vi "S2C_VLFT10_Proc_Commands.vi"(7 "VI_Ref":refnum<vi>, 8 "Error In":errorcluster, 10 "Settings":T1, 11 "Q-Ref":refnum<queue>) -> (0 "Error Out":errorcluster, 2 "Exit?":bool, 3 "Response":variant)   [LabVIEW 2015]
uses:
  S2C_VLFT10_Proc_Globals.vi
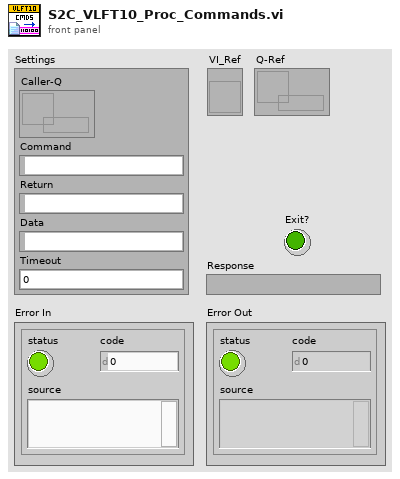
[diagram p1: front panel]
types:
  T1 = cluster{"Caller-Q":refnum<queue>, "Command":string, "Return":string, "Data":variant, "Timeout":dbl}
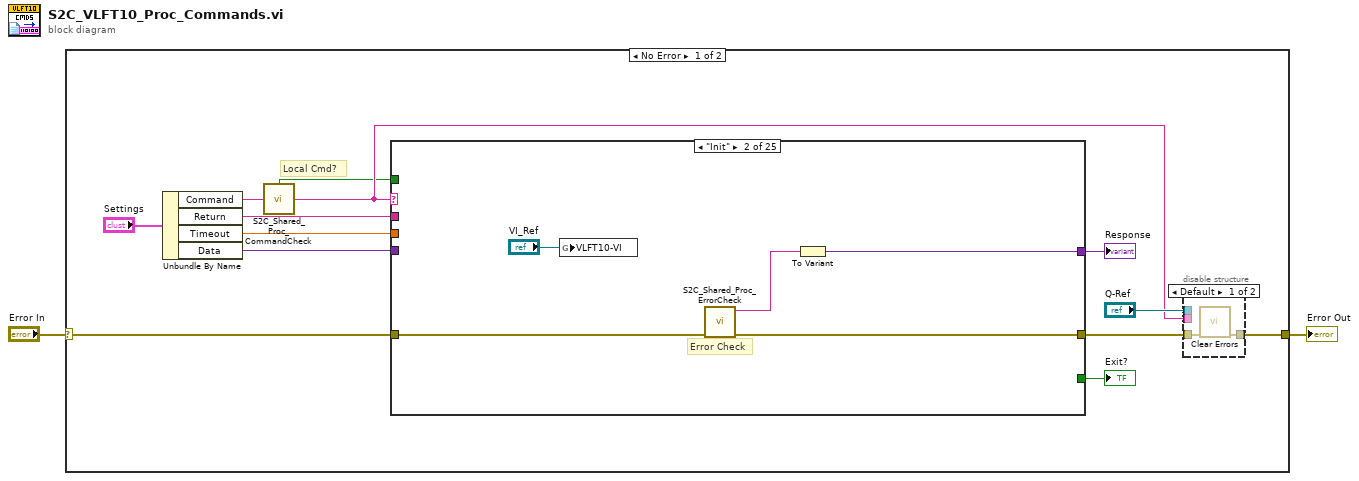
[diagram p0: block diagram]
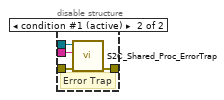
[diagram p2: hidden frame]
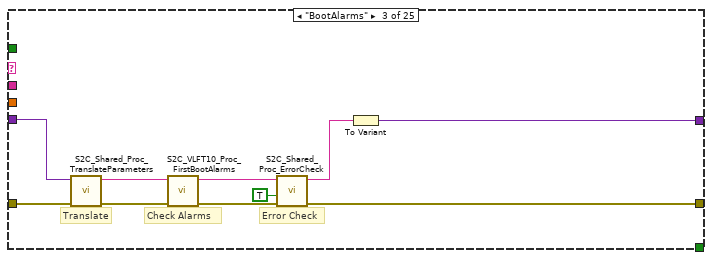
[diagram p4: hidden frame]
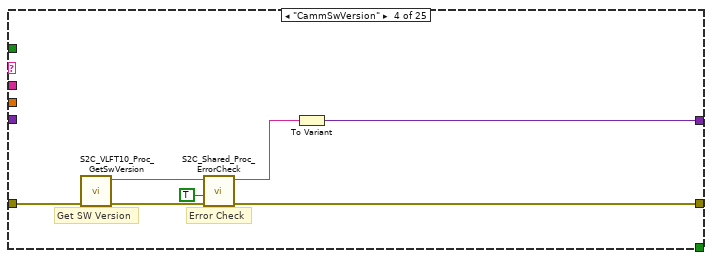
[diagram p5: hidden frame]
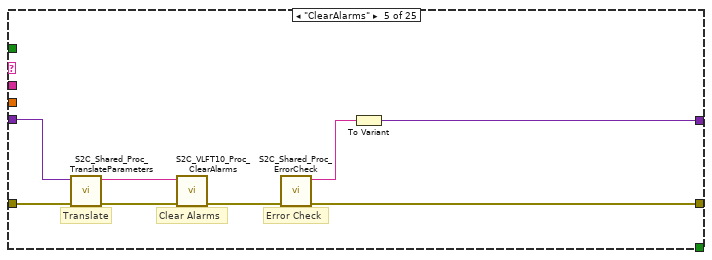
[diagram p6: hidden frame]
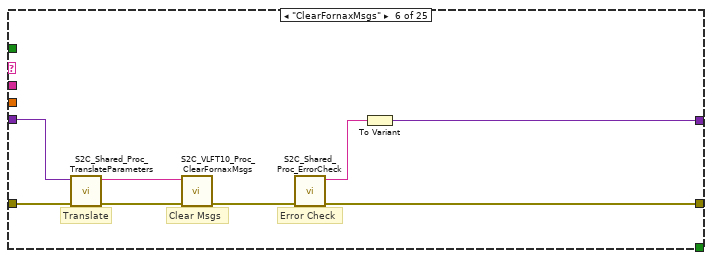
[diagram p7: hidden frame]
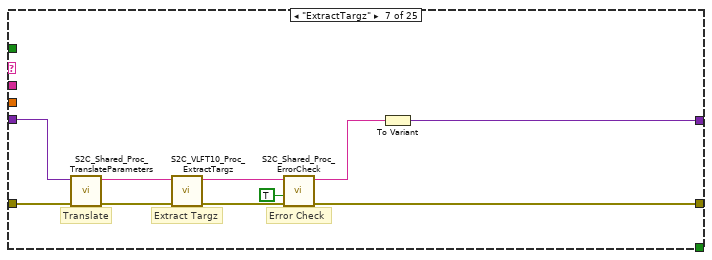
[diagram p8: hidden frame]
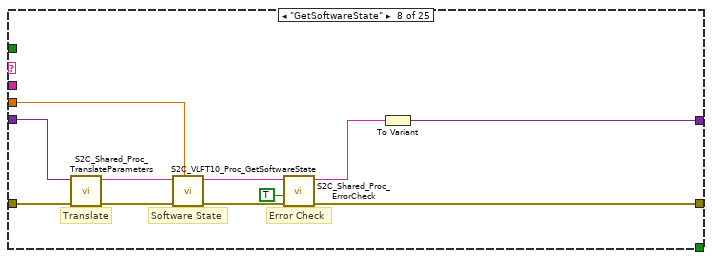
[diagram p9: hidden frame]
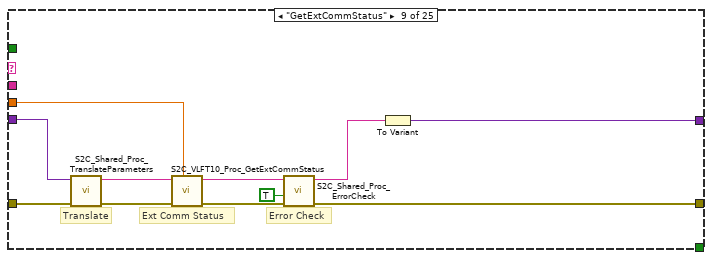
[diagram p10: hidden frame]
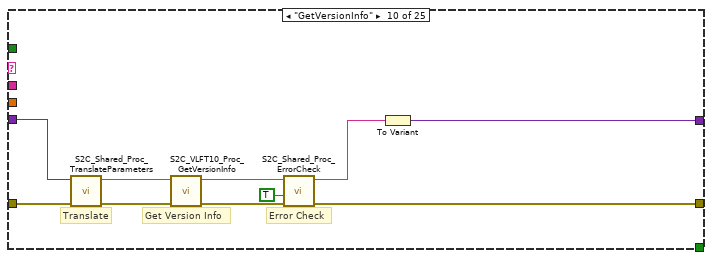
[diagram p11: hidden frame]
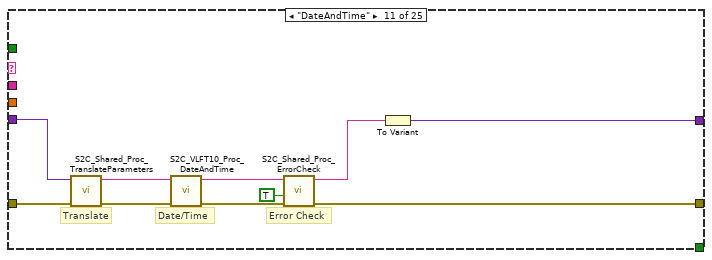
[diagram p12: hidden frame]
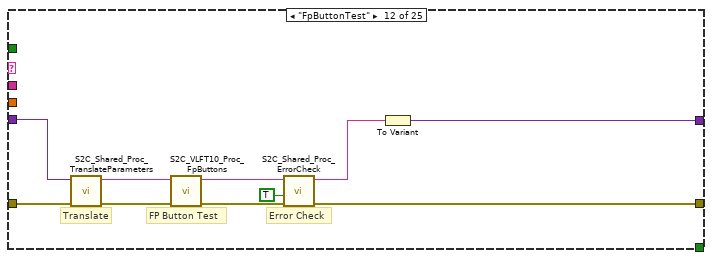
[diagram p13: hidden frame]
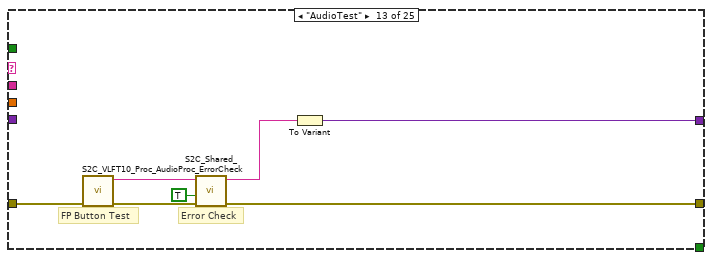
[diagram p14: hidden frame]
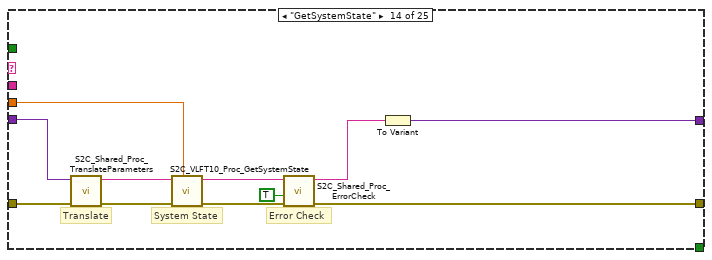
[diagram p15: hidden frame]
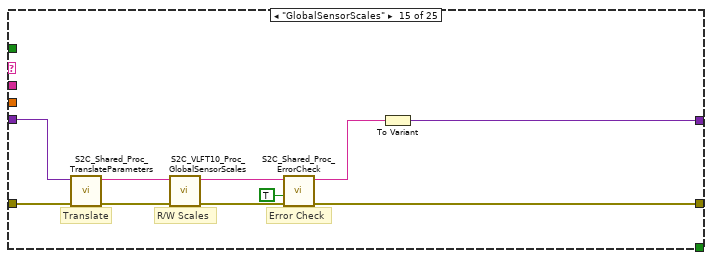
[diagram p16: hidden frame]
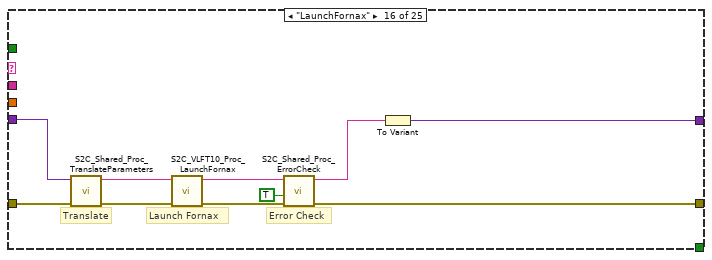
[diagram p17: hidden frame]
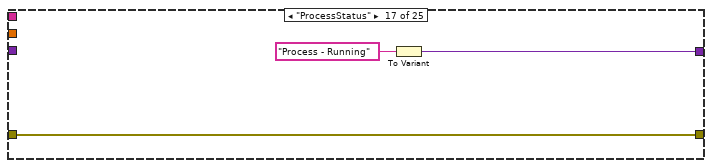
[diagram p18: hidden frame]
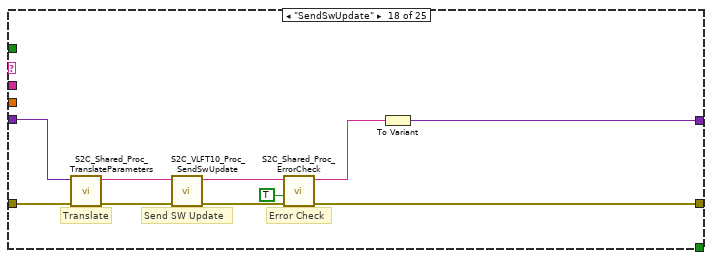
[diagram p19: hidden frame]
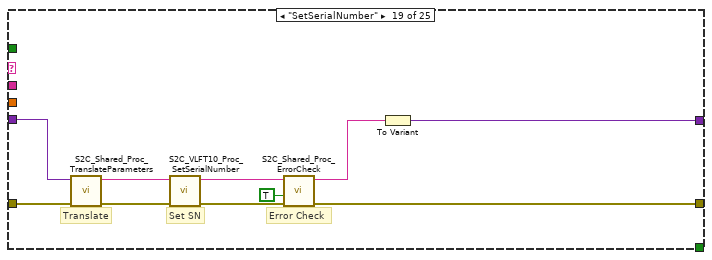
[diagram p20: hidden frame]
diagram:
  n1 = case shown="No Error" "Error In" {
    selector: "Error In" -> [w15 w237]
    tunnel: [w6 w236] -> w1
    frame No Error {
      # "Local Cmd?"
      n2 = Unbundle By Name("Settings") -> ("Command"=w5:string, "Return"=w12:string, "Timeout"=w10:dbl, "Data"=w11:variant)
      n3 = call "S2C_Shared_Proc_CommandCheck.vi"("Cmd In"=w5) -> ("Local?"=w3:bool, "Cmd Out"=w4:string)  [unwired: 13 in]
      n4 = case shown="\"Init\"" w4 {
        tunnel: w15 -> [w22 w23 w36 w39 w49 w57 w64 w75 w86 w96 w106 w116 w123 w134 w144 w154 w161 w167 w177 w187 w197 w208 w215 w225 w232]
        tunnel: [w22 w25 w28 w38 w50 w60 w65 w76 w87 w97 w107 w117 w124 w135 w145 w155 w161 w168 w178 w188 w198 w209 w216 w224 w227] -> w7
        tunnel: [_ w26 w37 w43 w51 w58 w70 w81 w92 w102 w112 w122 w129 w140 w150 w160 w163 w173 w183 w193 w203 w214 w221 _ w233] -> w14
        tunnel: w12 -> [_ _ _ _ _ _ _ _ _ _ _ _ _ _ _ _ _ _ _ _ _ _ _ _ _]
        tunnel: w11 -> [_ _ w35 _ w48 w53 w63 w74 w85 w95 w105 w115 _ w133 w143 w153 _ w166 w176 w186 w196 w207 _ w223 _]
        tunnel: w10 -> [_ _ _ _ _ _ _ w71 w82 _ _ _ _ w130 _ _ _ _ _ _ _ w204 _ _ _]
        tunnel: w3 -> [_ _ _ _ _ _ _ _ _ _ _ _ _ _ _ _ _ _ _ _ _ _ _ w222 _]
        tunnel: [_ _ _ _ _ _ _ _ _ _ _ _ _ _ _ _ _ _ _ _ _ _ _ _ TRUE] -> w9
        frame "Other", Default {
        }
        frame "Init" {
          # "Error Check"
          n5 = global write "S2C_VLFT10_Proc_Globals.vi" "VLFT10-VI"("VI_Ref") -> ()
          n6 = call "S2C_Shared_Proc_ErrorCheck.vi"("Error In"=w23) -> ("Error Out"=w25:errorcluster, "Status"=w27:string)  [unwired: 9 in]
          n7 = To Variant(anything=w27) -> (Variant=w26:variant)
        }
        frame "BootAlarms" {
          # "Check Alarms"
          # "Error Check"
          # "Translate"
          n8 = call "S2C_Shared_Proc_TranslateParameters.vi"("Error In"=w36, "Data"=w35) -> ("Error Out"=w30:errorcluster, "JSON Cluster"=w29:string)  [unwired: 8 in]
          n9 = call "S2C_VLFT10_Proc_FirstBootAlarms.vi"("Error In"=w30, "Exceptions"=w29) -> ("Error Out"=w33:errorcluster, "Pass?"=w32:string)  [unwired: 8 in]
          n10 = call "S2C_Shared_Proc_ErrorCheck.vi"("Error In"=w33, "ExpReply?"=TRUE, "Reply Text"=w32) -> ("Error Out"=w28:errorcluster, "Status"=w34:string)  [unwired: 7 in]
          n11 = To Variant(anything=w34) -> (Variant=w37:variant)
        }
        frame "CammSwVersion" {
          # "Get SW Version"
          # "Error Check"
          n12 = call "S2C_VLFT10_Proc_GetSwVersion.vi"("Error In"=w39) -> ("Error Out"=w42:errorcluster, "ItemValue"=w41:string)  [unwired: 8 in, 1 out]
          n13 = call "S2C_Shared_Proc_ErrorCheck.vi"("Error In"=w42, "ExpReply?"=TRUE, "Reply Text"=w41) -> ("Error Out"=w38:errorcluster, "Status"=w44:string)  [unwired: 7 in]
          n14 = To Variant(anything=w44) -> (Variant=w43:variant)
        }
        frame "ClearAlarms" {
          # "Clear Alarms"
          # "Translate"
          # "Error Check"
          n15 = call "S2C_Shared_Proc_TranslateParameters.vi"("Error In"=w49, "Data"=w48) -> ("Error Out"=w47:errorcluster, "JSON Cluster"=w45:string)  [unwired: 8 in]
          n16 = call "S2C_VLFT10_Proc_ClearAlarms.vi"("Error In"=w47, "Alarms"=w45) -> ("Error Out"=w46:errorcluster)  [unwired: 9 in]
          n17 = call "S2C_Shared_Proc_ErrorCheck.vi"("Error In"=w46) -> ("Error Out"=w50:errorcluster, "Status"=w52:string)  [unwired: 9 in]
          n18 = To Variant(anything=w52) -> (Variant=w51:variant)
        }
        frame "ClearFornaxMsgs" {
          # "Clear Msgs"
          # "Translate"
          # "Error Check"
          n19 = call "S2C_Shared_Proc_TranslateParameters.vi"("Error In"=w57, "Data"=w53) -> ("Error Out"=w56:errorcluster, "JSON Cluster"=w54:string)  [unwired: 8 in]
          n20 = call "S2C_VLFT10_Proc_ClearFornaxMsgs.vi"("Error In"=w56, "ClearMsg"=w54) -> ("Error Out"=w55:errorcluster)  [unwired: 9 in]
          n21 = call "S2C_Shared_Proc_ErrorCheck.vi"("Error In"=w55) -> ("Error Out"=w60:errorcluster, "Status"=w59:string)  [unwired: 9 in]
          n22 = To Variant(anything=w59) -> (Variant=w58:variant)
        }
        frame "ExtractTargz" {
          # "Translate"
          # "Extract Targz"
          # "Error Check"
          n23 = call "S2C_Shared_Proc_TranslateParameters.vi"("Error In"=w64, "Data"=w63) -> ("Error Out"=w62:errorcluster, "JSON Cluster"=w61:string)  [unwired: 8 in]
          n24 = call "S2C_VLFT10_Proc_ExtractTargz.vi"("Error In"=w62, "Paths"=w61) -> ("Error Out"=w68:errorcluster, "Result"=w67:string)  [unwired: 8 in]
          n25 = call "S2C_Shared_Proc_ErrorCheck.vi"("Error In"=w68, "ExpReply?"=TRUE, "Reply Text"=w67) -> ("Error Out"=w65:errorcluster, "Status"=w69:string)  [unwired: 7 in]
          n26 = To Variant(anything=w69) -> (Variant=w70:variant)
        }
        frame "GetSoftwareState" {
          # "Translate"
          # "Software State"
          # "Error Check"
          n27 = call "S2C_Shared_Proc_TranslateParameters.vi"("Error In"=w75, "Data"=w74) -> ("Error Out"=w73:errorcluster, "JSON Cluster"=w72:string)  [unwired: 8 in]
          n28 = call "S2C_VLFT10_Proc_GetSoftwareState.vi"("Timeout"=w71, "Error In"=w73, "State"=w72) -> ("Error Out"=w79:errorcluster, "Result"=w78:string)  [unwired: 7 in]
          n29 = call "S2C_Shared_Proc_ErrorCheck.vi"("Error In"=w79, "ExpReply?"=TRUE, "Reply Text"=w78) -> ("Error Out"=w76:errorcluster, "Status"=w80:string)  [unwired: 7 in]
          n30 = To Variant(anything=w80) -> (Variant=w81:variant)
        }
        frame "GetExtCommStatus" {
          # "Translate"
          # "Ext Comm Status"
          # "Error Check"
          n31 = call "S2C_Shared_Proc_TranslateParameters.vi"("Error In"=w86, "Data"=w85) -> ("Error Out"=w84:errorcluster, "JSON Cluster"=w83:string)  [unwired: 8 in]
          n32 = call "S2C_VLFT10_Proc_GetExtCommStatus.vi"("Timeout"=w82, "Error In"=w84, "Status"=w83) -> ("Error Out"=w90:errorcluster, "Result"=w89:string)  [unwired: 7 in]
          n33 = call "S2C_Shared_Proc_ErrorCheck.vi"("Error In"=w90, "ExpReply?"=TRUE, "Reply Text"=w89) -> ("Error Out"=w87:errorcluster, "Status"=w91:string)  [unwired: 7 in]
          n34 = To Variant(anything=w91) -> (Variant=w92:variant)
        }
        frame "GetVersionInfo" {
          # "Translate"
          # "Get Version Info"
          # "Error Check"
          n35 = call "S2C_Shared_Proc_TranslateParameters.vi"("Error In"=w96, "Data"=w95) -> ("Error Out"=w94:errorcluster, "JSON Cluster"=w93:string)  [unwired: 8 in]
          n36 = call "S2C_VLFT10_Proc_GetVersionInfo.vi"("Error In"=w94, "Item"=w93) -> ("Error Out"=w100:errorcluster, "Value"=w99:string)  [unwired: 7 in, 1 out]
          n37 = call "S2C_Shared_Proc_ErrorCheck.vi"("Error In"=w100, "ExpReply?"=TRUE, "Reply Text"=w99) -> ("Error Out"=w97:errorcluster, "Status"=w101:string)  [unwired: 7 in]
          n38 = To Variant(anything=w101) -> (Variant=w102:variant)
        }
        frame "DateAndTime" {
          # "Translate"
          # "Date/Time"
          # "Error Check"
          n39 = call "S2C_Shared_Proc_TranslateParameters.vi"("Error In"=w106, "Data"=w105) -> ("Error Out"=w104:errorcluster, "JSON Cluster"=w103:string)  [unwired: 8 in]
          n40 = call "S2C_VLFT10_Proc_DateAndTime.vi"("Error In"=w104, "Time"=w103) -> ("Error Out"=w110:errorcluster, "Result"=w109:string)  [unwired: 8 in]
          n41 = call "S2C_Shared_Proc_ErrorCheck.vi"("Error In"=w110, "ExpReply?"=TRUE, "Reply Text"=w109) -> ("Error Out"=w107:errorcluster, "Status"=w111:string)  [unwired: 7 in]
          n42 = To Variant(anything=w111) -> (Variant=w112:variant)
        }
        frame "FpButtonTest" {
          # "Translate"
          # "FP Button Test"
          # "Error Check"
          n43 = call "S2C_Shared_Proc_TranslateParameters.vi"("Error In"=w116, "Data"=w115) -> ("Error Out"=w114:errorcluster, "JSON Cluster"=w113:string)  [unwired: 8 in]
          n44 = call "S2C_VLFT10_Proc_FpButtons.vi"("Error In"=w114, "Button"=w113) -> ("Error Out"=w120:errorcluster, "Result"=w119:string)  [unwired: 8 in]
          n45 = call "S2C_Shared_Proc_ErrorCheck.vi"("Error In"=w120, "ExpReply?"=TRUE, "Reply Text"=w119) -> ("Error Out"=w117:errorcluster, "Status"=w121:string)  [unwired: 7 in]
          n46 = To Variant(anything=w121) -> (Variant=w122:variant)
        }
        frame "AudioTest" {
          # "FP Button Test"
          # "Error Check"
          n47 = call "S2C_VLFT10_Proc_Audio.vi"("Error In"=w123) -> ("Error Out"=w127:errorcluster, "Result"=w126:string)  [unwired: 9 in]
          n48 = call "S2C_Shared_Proc_ErrorCheck.vi"("Error In"=w127, "ExpReply?"=TRUE, "Reply Text"=w126) -> ("Error Out"=w124:errorcluster, "Status"=w128:string)  [unwired: 7 in]
          n49 = To Variant(anything=w128) -> (Variant=w129:variant)
        }
        frame "GetSystemState" {
          # "Translate"
          # "System State"
          # "Error Check"
          n50 = call "S2C_Shared_Proc_TranslateParameters.vi"("Error In"=w134, "Data"=w133) -> ("Error Out"=w132:errorcluster, "JSON Cluster"=w131:string)  [unwired: 8 in]
          n51 = call "S2C_VLFT10_Proc_GetSystemState.vi"("Timeout"=w130, "Error In"=w132, "State"=w131) -> ("Error Out"=w138:errorcluster, "Result"=w137:string)  [unwired: 7 in]
          n52 = call "S2C_Shared_Proc_ErrorCheck.vi"("Error In"=w138, "ExpReply?"=TRUE, "Reply Text"=w137) -> ("Error Out"=w135:errorcluster, "Status"=w139:string)  [unwired: 7 in]
          n53 = To Variant(anything=w139) -> (Variant=w140:variant)
        }
        frame "GlobalSensorScales" {
          # "Translate"
          # "R/W Scales"
          # "Error Check"
          n54 = call "S2C_Shared_Proc_TranslateParameters.vi"("Error In"=w144, "Data"=w143) -> ("Error Out"=w142:errorcluster, "JSON Cluster"=w141:string)  [unwired: 8 in]
          n55 = call "S2C_VLFT10_Proc_GlobalSensorScales.vi"("Error In"=w142, "Scales"=w141) -> ("Error Out"=w148:errorcluster, "Result"=w147:string)  [unwired: 8 in]
          n56 = call "S2C_Shared_Proc_ErrorCheck.vi"("Error In"=w148, "ExpReply?"=TRUE, "Reply Text"=w147) -> ("Error Out"=w145:errorcluster, "Status"=w149:string)  [unwired: 7 in]
          n57 = To Variant(anything=w149) -> (Variant=w150:variant)
        }
        frame "LaunchFornax" {
          # "Translate"
          # "Launch Fornax"
          # "Error Check"
          n58 = call "S2C_Shared_Proc_TranslateParameters.vi"("Error In"=w154, "Data"=w153) -> ("Error Out"=w152:errorcluster, "JSON Cluster"=w151:string)  [unwired: 8 in]
          n59 = call "S2C_VLFT10_Proc_LaunchFornax.vi"("Error In"=w152, "Selection"=w151) -> ("Error Out"=w158:errorcluster, "Version"=w157:string)  [unwired: 8 in]
          n60 = call "S2C_Shared_Proc_ErrorCheck.vi"("Error In"=w158, "ExpReply?"=TRUE, "Reply Text"=w157) -> ("Error Out"=w155:errorcluster, "Status"=w159:string)  [unwired: 7 in]
          n61 = To Variant(anything=w159) -> (Variant=w160:variant)
        }
        frame "ProcessStatus" {
          n62 = To Variant(anything="Process - Running") -> (Variant=w163:variant)
        }
        frame "SendSwUpdate" {
          # "Translate"
          # "Send SW Update"
          # "Error Check"
          n63 = call "S2C_Shared_Proc_TranslateParameters.vi"("Error In"=w167, "Data"=w166) -> ("Error Out"=w165:errorcluster, "JSON Cluster"=w164:string)  [unwired: 8 in]
          n64 = call "S2C_VLFT10_Proc_SendSwUpdate.vi"("Error In"=w165, "Paths"=w164) -> ("Error Out"=w171:errorcluster, "Result"=w170:string)  [unwired: 8 in]
          n65 = call "S2C_Shared_Proc_ErrorCheck.vi"("Error In"=w171, "ExpReply?"=TRUE, "Reply Text"=w170) -> ("Error Out"=w168:errorcluster, "Status"=w172:string)  [unwired: 7 in]
          n66 = To Variant(anything=w172) -> (Variant=w173:variant)
        }
        frame "SetSerialNumber" {
          # "Translate"
          # "Set SN"
          # "Error Check"
          n67 = call "S2C_Shared_Proc_TranslateParameters.vi"("Error In"=w177, "Data"=w176) -> ("Error Out"=w175:errorcluster, "JSON Cluster"=w174:string)  [unwired: 8 in]
          n68 = call "S2C_VLFT10_Proc_SetSerialNumber.vi"("Error In"=w175, "SN In"=w174) -> ("Error Out"=w181:errorcluster, "Result"=w180:string)  [unwired: 8 in]
          n69 = call "S2C_Shared_Proc_ErrorCheck.vi"("Error In"=w181, "ExpReply?"=TRUE, "Reply Text"=w180) -> ("Error Out"=w178:errorcluster, "Status"=w182:string)  [unwired: 7 in]
          n70 = To Variant(anything=w182) -> (Variant=w183:variant)
        }
        frame "TriverseSliderSelect" {
          # "Translate"
          # "Set Slider"
          # "Error Check"
          n71 = call "S2C_Shared_Proc_TranslateParameters.vi"("Error In"=w187, "Data"=w186) -> ("Error Out"=w185:errorcluster, "JSON Cluster"=w184:string)  [unwired: 8 in]
          n72 = call "S2C_VLFT10_Proc_TriverseSliderSelect.vi"("Error In"=w185, "SliderSelect"=w184) -> ("Error Out"=w191:errorcluster, "Result"=w190:string)  [unwired: 8 in]
          n73 = call "S2C_Shared_Proc_ErrorCheck.vi"("Error In"=w191, "ExpReply?"=TRUE, "Reply Text"=w190) -> ("Error Out"=w188:errorcluster, "Status"=w192:string)  [unwired: 7 in]
          n74 = To Variant(anything=w192) -> (Variant=w193:variant)
        }
        frame "RfPaths" {
          # "Translate"
          # "Set Paths"
          # "Error Check"
          n75 = call "S2C_Shared_Proc_TranslateParameters.vi"("Error In"=w197, "Data"=w196) -> ("Error Out"=w195:errorcluster, "JSON Cluster"=w194:string)  [unwired: 8 in]
          n76 = call "S2C_VLFT10_Proc_RfPaths.vi"("Error In"=w195, "HandSwitch"=w194) -> ("Error Out"=w201:errorcluster, "Result"=w200:string)  [unwired: 8 in]
          n77 = call "S2C_Shared_Proc_ErrorCheck.vi"("Error In"=w201, "ExpReply?"=TRUE, "Reply Text"=w200) -> ("Error Out"=w198:errorcluster, "Status"=w202:string)  [unwired: 7 in]
          n78 = To Variant(anything=w202) -> (Variant=w203:variant)
        }
        frame "WaitForReboot" {
          # "Translate"
          # "Reboot Wait"
          # "Error Check"
          n79 = call "S2C_Shared_Proc_TranslateParameters.vi"("Error In"=w208, "Data"=w207) -> ("Error Out"=w206:errorcluster, "JSON Cluster"=w205:string)  [unwired: 8 in]
          n80 = call "S2C_VLFT10_Proc_WaitForReboot.vi"("Timeout"=w204, "Error In"=w206, "State"=w205) -> ("Error Out"=w212:errorcluster, "Result"=w211:string)  [unwired: 7 in]
          n81 = call "S2C_Shared_Proc_ErrorCheck.vi"("Error In"=w212, "ExpReply?"=TRUE, "Reply Text"=w211) -> ("Error Out"=w209:errorcluster, "Status"=w213:string)  [unwired: 7 in]
          n82 = To Variant(anything=w213) -> (Variant=w214:variant)
        }
        frame "WaitForRebootReset" {
          # "Reboot Wait"
          # "Error Check"
          n83 = call "S2C_VLFT10_Proc_WaitForRebootReset.vi"("Error In"=w215) -> ("Error Out"=w219:errorcluster, "Result"=w218:string)  [unwired: 9 in]
          n84 = call "S2C_Shared_Proc_ErrorCheck.vi"("Error In"=w219, "ExpReply?"=TRUE, "Reply Text"=w218) -> ("Error Out"=w216:errorcluster, "Status"=w220:string)  [unwired: 7 in]
          n85 = To Variant(anything=w220) -> (Variant=w221:variant)
        }
        frame "Error" {
          # "Manage Error"
          n86 = call "S2C_Shared_Proc_ManageError.vi"("Local?"=w222, "Process"="VLFT10", "Error In"=w225, "Data"=w223) -> ("Error Out"=w224:errorcluster)  [unwired: 7 in]
        }
        frame "Exit" {
          # "Release Q"
          # "Clear Error"
          # "Error Check"
          n87 = local read "Q-Ref"() -> (w230:refnum<queue>)
          n88 = Release Queue(queue=w230, force destroy? (F)=TRUE, error in (no error)=w232) -> (error out=w231:errorcluster)  [unwired: 2 out]
          n89 = call "S2C_Shared_Proc_ErrorCheck.vi"("Error In"=w231) -> ("Error Out"=w228:errorcluster, "Status"=w234:string)  [unwired: 9 in]
          n90 = To Variant(anything=w234) -> (Variant=w233:variant)
          n91 = call <vilib>:"Clear Errors.vi"("error in (no error)"=w228) -> ("error out"=w227:errorcluster)  [unwired: 5 in, 1 out]
        }
      }
      "Response" <- w14
      "Exit?" <- w9
      n92 = disable-structure shown="Default" {
        disable-tunnel: w7 -> [w17 w21]
        disable-tunnel: [w16 w20] -> w6
        disable-tunnel: w4 -> [_ w19]
        disable-tunnel: "Q-Ref" -> [_ w18]
        frame condition #0 {
          n93 = call <vilib>:"Clear Errors.vi"("error in (no error)"=w17) -> ("error out"=w16:errorcluster)  [unwired: 5 in, 1 out]
        }
        frame condition #1 (active) {
          # "Error Trap"
          n94 = call "S2C_Shared_Proc_ErrorTrap.vi"("Error In"=w21, "Command"=w19, "Q-Ref"=w18) -> ("Error Out"=w20:errorcluster)  [unwired: 8 in]
        }
      }
    }
    frame Error {
      # "Clear Error"
      # "Manage Error"
      n95 = Bundle("Dequeue Element", "error IO"=w237) -> (w241:cluster{string, "error IO":errorcluster})  [unwired: 1 in]
      n96 = call <vilib>:"Clear Errors.vi"("error in (no error)"=w237) -> ("error out"=w238:errorcluster)  [unwired: 5 in, 1 out]
      n97 = To Variant(anything=w241) -> (Variant=w239:variant)
      n98 = call "S2C_Shared_Proc_ManageError.vi"("Process"="Fornax", "Error In"=w238, "Data"=w239) -> ("Error Out"=w236:errorcluster)  [unwired: 8 in]
    }
  }
  "Error Out" <- w1
